vi "Get Data I16.vi"(8 "error in (no error)":errorcluster, 11 "DAQmx Digitizer in":refnum<class "DAQmx Digitizer.lvclass">) -> (0 "error out":errorcluster, 1 "Current read position":i32, 2 "data":i16[][](array[numeric]), 3 "DAQmx Digitizer out":refnum<class "DAQmx Digitizer.lvclass">, 4 "Finished":bool)   [LabVIEW 2015, in "DAQmx Digitizer.lvclass"]
uses:
  DAQmx Digitizer.lvclass
  Instruments/Pulse Driver/Pulse Driver.lvclass/Pulse Driver.ctl
  DAQmx Digitizer.lvclass/DAQmx Digitizer.ctl
  <vilib>/DAQmx/read.llb/DAQmx Read (Analog 2D I16 NChan NSamp).vi
  Instruments/Pulse Driver/Read Current read position.vi
  Instruments/Pulse Driver/Read Samples per channel.vi
  Instruments/Pulse Driver/Read Samples per read.vi
  <vilib>/DAQmx/miscellaneous.llb/DAQmx Fill In Error Info.vi
  <resource>/objmgr/daqmx.rc
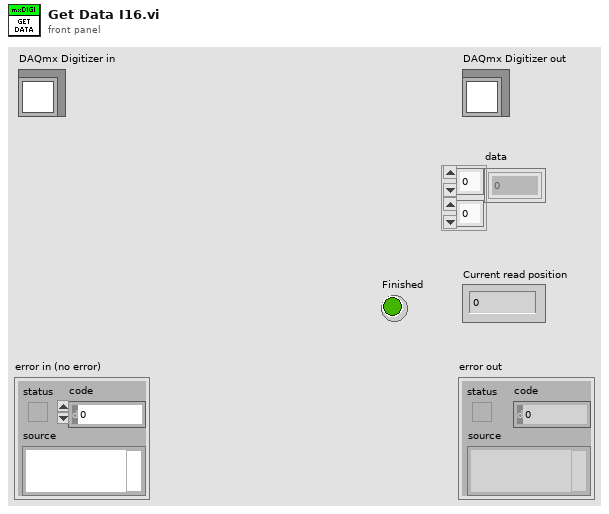
[diagram p1: front panel]
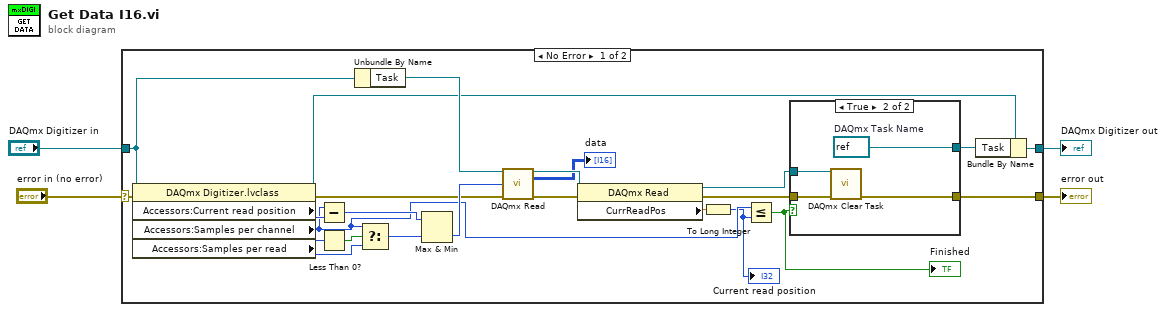
[diagram p0: block diagram]
diagram:
  n1 = case shown="No Error" "error in (no error)" {
    selector: "error in (no error)" -> [w8 w35]
    tunnel: [w16 w35] -> w3
    tunnel: [w12 w34] -> w1
    tunnel: "DAQmx Digitizer in" -> [w27 w34]
    frame No Error {
      n2 = property class="DAQmx Digitizer.lvclass"(reference=w27, error in=w8) -> (reference out=w13:refnum<class "DAQmx Digitizer.lvclass">, error out=w7:errorcluster, "Accessors:Current read position"=w11:i32, "Accessors:Samples per channel"=w10:i32, "Accessors:Samples per read"=w6:i32)
      n3 = Subtract(x=w10, y=w11) -> (x-y=w26:i32)
      n4 = Less Than 0?(x=w6) -> (x < 0?=w15:bool)
      n5 = Unbundle By Name(w27) -> ("Task"=w25:refnum<k21>)
      n6 = Select(t=w10, s=w15, f=w6) -> (s? t:f=w14:i32)
      n7 = Max & Min(x=w26, y=w14) -> (min(x,y)=w24:i32)  [unwired: 1 out]
      n8 = call-poly <vilib>:"DAQmx Read.vi"("task/channels in"=w25, "number of samples per channel"=w24, "error in"=w7) -> ("task out"=w23:refnum<k21>, "data"=→"data":i16[][], "error out"=w22:errorcluster)  [unwired: 1 in, 9 out]
      n9 = property class="DAQmx Read"(reference=w23, error in=w22) -> (reference out=w18:refnum<k21>, error out=w19:errorcluster, "CurrReadPos"=w20:dbl)
      n10 = To Long Integer(number=w20) -> (32bit integer=w9:i32)
      "Current read position" <- w9
      n11 = Less Or Equal?(x=w10, y=w9) -> (x <= y?=w5:bool)
      "Finished" <- w5
      n12 = case shown="True" w5 {
        tunnel: [w29 w33] -> w16
        tunnel: w18 -> [w28 w31]
        tunnel: w19 -> [w29 w32]
        tunnel: [w28 w30] -> w17
        frame False {
        }
        frame True {
          w30 = refnum<k21> refnum  # DAQmx Task Name
          n13 = call <vilib>:"DAQmx Clear Task.vi"("task in"=w31, "error in"=w32) -> ("error out"=w33:errorcluster)  [unwired: 13 out]
        }
      }
      n14 = Bundle By Name(cluster=w13, "Task"=w17) -> (w12:refnum<class "DAQmx Digitizer.lvclass">)
    }
    frame Error {
    }
  }
  "error out" <- w3
  "DAQmx Digitizer out" <- w1
